vi "Ballard XML Generator.Params Instructions.vi"(11 "string in":string) -> (3 "string out":string)   [LabVIEW 2017]
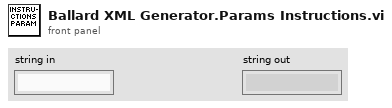
[diagram p1: front panel]
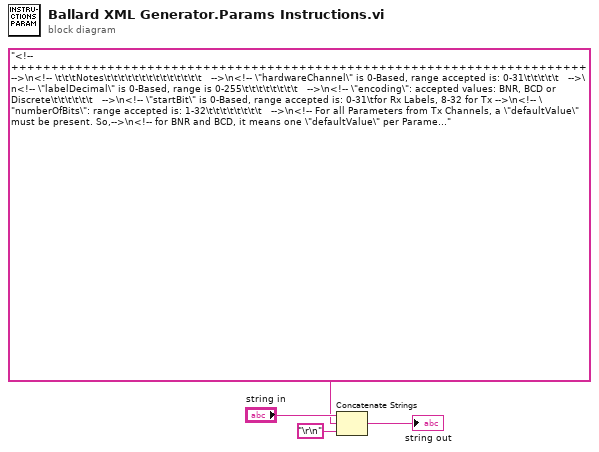
[diagram p0: block diagram]
diagram:
  n1 = Concatenate Strings("string in", "<!-- ++++++++++++++++++++++++++++++++++++++++++++++++++++++++++++++++++++++++  -->\n<!-- \t\t\tNotes\t\t\t\t\t\t\t\t\t\t\t\t\t\t   -->\n<!-- \"hardwareChannel\" is 0-Based, range accepted is: 0-31\t\t\t\t\t   -->\n<!-- \"labelDecimal\" is 0-Based, range is 0-255\t\t\t\t\t\t\t\t   -->\n<!-- \"encoding\": accepted values: BNR, BCD or Discrete\t\t\t\t\t\t   -->\n<!-- \"startBit\" is 0-Based, range accepted is: 0-31\tfor Rx Labels, 8-32 for Tx -->\n<!-- \"numberOfBits\": range accepted is: 1-32\t\t\t\t\t\t\t\t   -->\n<!-- For all Parameters from Tx Channels, a \"defaultValue\" must be present. So,-->\n<!-- for BNR and BCD, it means one \"defaultValue\" per Parameter, for Discrete  -->\n<!-- it means one \"defaultValue\" instance per bit of the Parameter. \t\t   -->\n<!--             \t\t\t\t\t\t\t\t\t\t\t\t\t\t\t   -->\n<!-- For Discrete encoding Parameter, for defaultValue, 0 value is considered  -->\n<!-- \"false\", any value different from 0 is considered \"true\".\t\t\t\t   -->\n<!--             \t\t\t\t\t\t\t\t\t\t\t\t\t\t\t   -->\n<!-- For BCD \"encoding\", if signed is true, we assume that sign information is -->\n<!-- stored in SSM Bits with following table: 00: positive , 11: negative.\t   -->\n<!-- For \"Discrete\" encoding type, there should be one name element per        -->\n<!-- numberOfBits of the Parameter.\t\t\t\t\t\t\t\t\t\t\t   -->\n<!-- For BCD encoding, \"numberOfBits\" includes only sum of bits used to encode -->\n<!-- digits, bits used to encode sign are excluded from that count. \t\t   -->\n<!-- For BCD encoding, \"startBit\" values supported are: 10, 14, 18, 22, 26.\t   -->\n<!-- ++++++++++++++++++++++++++++++++++++++++++++++++++++++++++++++++++++++++  -->", "\r\n") -> (→"string out":string)
